vi "AlazarCoprocessorDownload.vi"(3 "error in (no error)":errorcluster, 4 "Options":u32(ring) items=["None", "DMA Download"], 5 "File Name":string, 6 "Handle":u64) -> (0 "error out":errorcluster, 1 "Return Code":u32, 2 "Handle":u64)   [LabVIEW 2018]
doc: "Download an FPGA image in RBF (raw binary file) format to the coprocessor FPGA."
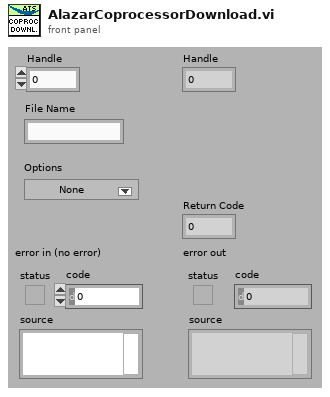
[diagram p1: front panel]
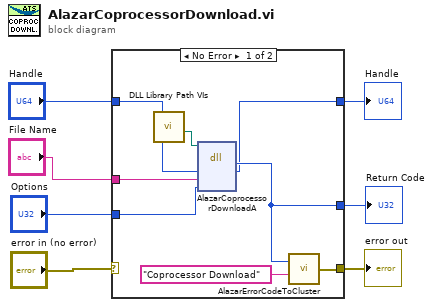
[diagram p0: block diagram]
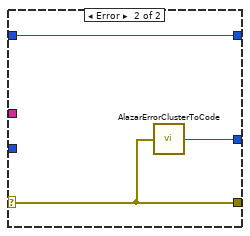
[diagram p2: hidden frame]
diagram:
  n1 = case shown="No Error" "error in (no error)" {
    selector: "error in (no error)" -> [_ w18]
    tunnel: [w12 w18] -> w6
    tunnel: [w14 w17] -> w5
    tunnel: "Handle" -> [w15 w16]
    tunnel: [w11 w16] -> w3
    tunnel: "File Name" -> [w10 _]
    tunnel: "Options" -> [w9 _]
    frame No Error {
      n2 = call "DLL Library Path VIs.vi"() -> ("Alazar"=w8:path)  [unwired: 9 in, 2 out]
      n3 = dll-call lib="C:/Project/SerialSectOCT - FFT GPU/SerialSectOCT/Labview Software/DLL/ATSApi.dll" fn="AlazarCoprocessorDownloadA"(path in=w8, "handle"=w15, "fileName"=w10, "options"=w9) -> ("return type"=w14:u32, "handle"=w11:u64)  [unwired: 4 in, 2 out]
      n4 = call "AlazarErrorCodeToCluster.vi"("Message"="Coprocessor Download", "Error Code"=w14) -> ("error out"=w12:errorcluster)
    }
    frame Error {
      n5 = call "AlazarErrorClusterToCode.vi"("error in (no error)"=w18) -> ("Error Code"=w17:u32)
    }
  }
  "Handle" <- w3
  "error out" <- w6
  "Return Code" <- w5
